vi "upgrade_fault_branch.vi"(8 "Fault type":string="BCG", 9 "Event type":string="CL", 10 "node":i32, 11 "R fault":dbl) -> (3 "Result":string)   [LabVIEW 2020]
panel:
  # "1) RESISTÊNCIA DE FALTA\n2) RESISTÊNCIA FIXA ENTRE A CHAVE E O TERRA\n3) RC DE AMORTECIMENDO P FALTA DE CIRCUITO ABETO"
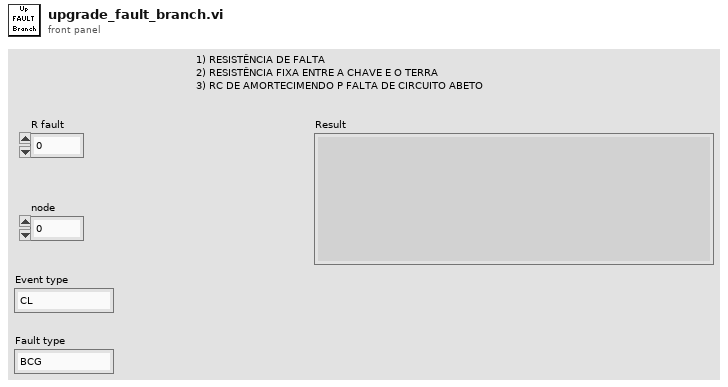
[diagram p1: front panel]
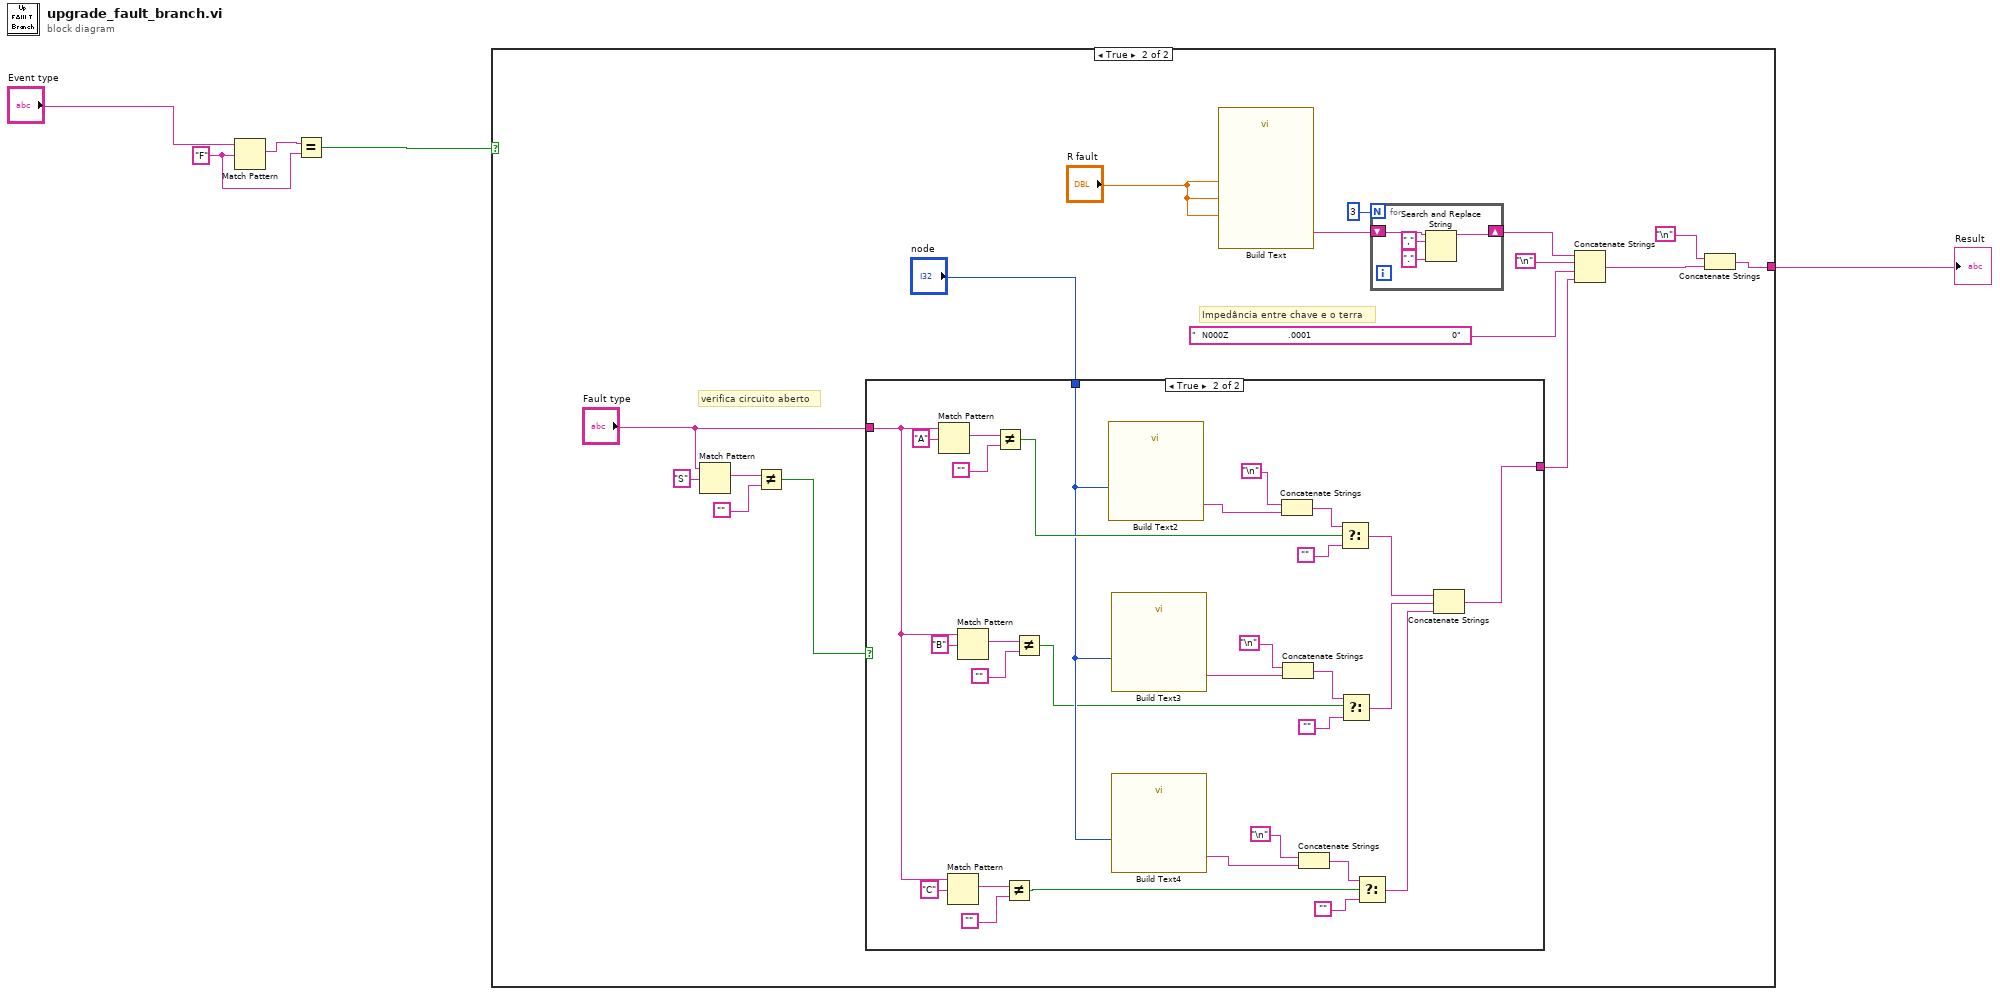
[diagram p0: block diagram]
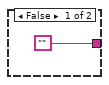
[diagram p3: hidden frame]
diagram:
  w4 = "F" ("regular expression")
  n1 = Match Pattern(string="Event type", regular expression=w4) -> (match substring=w3:string)  [unwired: 1 in, 3 out]
  n2 = Equal?(x=w3, y=w4) -> (x = y?=w1:bool)
  n3 = case shown="True" w1 {
    tunnel: [_ w7] -> w5
    frame False {
    }
    frame True {
      # "verifica circuito aberto"
      # "Impedância entre chave e o terra"
      n4 = Match Pattern(string="Fault type", regular expression="S") -> (match substring=w14:string)  [unwired: 1 in, 3 out]
      n5 = Not Equal?(x=w14, y="") -> (x != y?=w12:bool)
      n6 = case shown="True" w12 {
        tunnel: "Fault type" -> [_ w43]
        tunnel: ["" w39] -> w10
        tunnel: "node" -> [_ w40]
        frame False {
        }
        frame True {
          n7 = Match Pattern(string=w43, regular expression="A") -> (match substring=w51:string)  [unwired: 1 in, 3 out]
          n8 = Match Pattern(string=w43, regular expression="C") -> (match substring=w45:string)  [unwired: 1 in, 3 out]
          n9 = Match Pattern(string=w43, regular expression="B") -> (match substring=w48:string)  [unwired: 1 in, 3 out]
          n10 = Not Equal?(x=w51, y="") -> (x != y?=w42:bool)
          n11 = Not Equal?(x=w45, y="") -> (x != y?=w30:bool)
          n12 = Not Equal?(x=w48, y="") -> (x != y?=w33:bool)
          n13 = call "Build Text2"("node_A"=w40) -> ("Result"=w28:string)  [unwired: 13 in, 1 out]
          n14 = call "Build Text3"("node_B"=w40) -> ("Result"=w25:string)  [unwired: 13 in, 1 out]
          n15 = call "Build Text4"("node_C"=w40) -> ("Result"=w24:string)  [unwired: 13 in, 1 out]
          n16 = Concatenate Strings("\n", w28) -> (w38:string)
          n17 = Concatenate Strings("\n", w25) -> (w35:string)
          n18 = Concatenate Strings("\n", w24) -> (w32:string)
          n19 = Select(t=w38, s=w42, f="") -> (s? t:f=w37:string)
          n20 = Select(t=w35, s=w33, f="") -> (s? t:f=w34:string)
          n21 = Select(t=w32, s=w30, f="") -> (s? t:f=w29:string)
          n22 = Concatenate Strings(w37, w34, w29) -> (w39:string)
        }
      }
      n23 = call "Build Text"("R_a"="R fault", "R_b"="R fault", "R_c"="R fault") -> ("Result"=w20:string)  [unwired: 11 in, 1 out]
      n24 = for {
        N: 3 -> [_]
        shift-right: [w53] -> w19
        shift-left: w20 -> [w54]
        n25 = Search and Replace String(input string=w54, search string=",", replace string="." ("replace string (\"\")")) -> (result string=w53:string)  [unwired: 5 in, 3 out]
      }
      n26 = Concatenate Strings(w19, "\n", "  N000Z                    .0001                                               0", w10) -> (w8:string)
      n27 = Concatenate Strings("\n", w8) -> (w7:string)
    }
  }
  "Result" <- w5
